vi "myRIO v1.0 Timer IRQ Info FGV.vi"(7 "Action":T1=enum."Set", 8 "error in (no error)":errorcluster, 11 "Timer IRQ Array in":T2) -> (0 "error out":errorcluster, 3 "Timer IRQ Array out":T2)   [LabVIEW 2021]
uses:
  <vilib>/myRIO/Common/Instrument Driver Framework/myRIO v1.0/IRQ/typedefs/Timer IRQ Array.ctl
  <vilib>/myRIO/Common/Instrument Driver Framework/myRIO v1.0/IRQ/typedefs/Timer IRQ.ctl
  <vilib>/myRIO/Common/Instrument Driver Framework/myRIO v1.0/IRQ/typedefs/Callback VI Ref.ctl
  <vilib>/myRIO/Common/Instrument Driver Framework/Utilities/typedefs/FPGA Ref Manager Action Enum.ctl
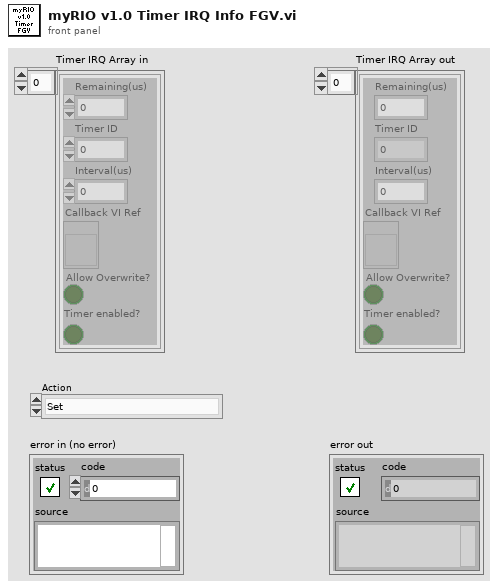
[diagram p1: front panel]
types:
  T1 = typedef "FPGA Ref Manager Action Enum.ctl" = enum16{"Get", "Set", "Reset"}
  T2 = typedef "Timer IRQ Array.ctl" = T3[]
  T3 = typedef "Timer IRQ.ctl" = cluster{"Remaining(us)":u32, "Timer ID":u8, "Interval(us)":u32, "Callback VI Ref":T4, "Allow Overwrite?":bool, "Timer enabled?":bool}
  T4 = typedef "Callback VI Ref.ctl" = refnum<vi>
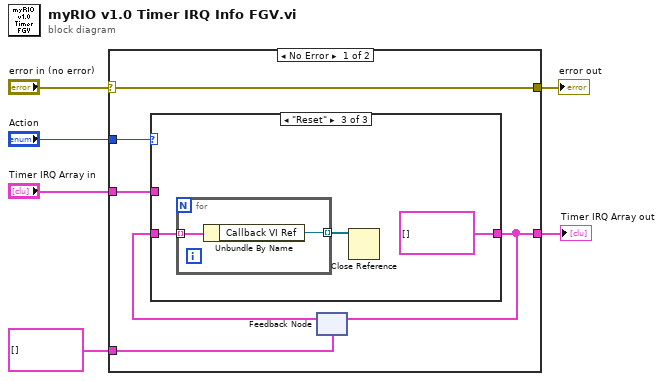
[diagram p0: block diagram]
diagram:
  n1 = case shown="No Error" "error in (no error)" {
    selector: "error in (no error)" -> [w8 w21]
    tunnel: "Action" -> [w12 _]
    tunnel: "Timer IRQ Array in" -> [w11 _]
    tunnel: [w10 w20] -> w4
    tunnel: [w8 w21] -> w2
    tunnel: T2 [] ("Interrupt Infos out") -> [w7 w20]
    frame No Error {
      n2 = feedback #1(w7) -> (w9:T2)
      n3 = case shown="\"Reset\"" w12 {
        tunnel: [w13 w14 T2 [] ("Interrupt Infos out")] -> w10
        tunnel: w11 -> [_ w14 _]
        tunnel: w9 -> [w13 _ w15]
        frame "Get", Default {
        }
        frame "Set" {
        }
        frame "Reset" {
          n4 = for {
            tunnel: w15 -> [w19] mode=indexing
            tunnel: [w18] -> w16 mode=indexing
            n5 = Unbundle By Name(w19) -> ("Callback VI Ref"=w18:T4)
          }
          n6 = Close Reference(reference=w16) -> ()  [unwired: 1 in, 1 out]
        }
      }
      n7 = feedback-in #1(w10) -> ()
    }
    frame Error {
    }
  }
  "Timer IRQ Array out" <- w4
  "error out" <- w2
